vi "create.vi"(5 "Reference":string, 6 "Balance":dbl, 7 "Date":timestamp, 8 "error in (no error)":errorcluster, 9 "Category":string, 10 "Description":string, 11 "Amount":dbl) -> (0 "error out":errorcluster, 3 "Banking Transaction out":refnum<class "Banking Transaction.lvclass">)   [LabVIEW 2018, in "Banking Transaction.lvclass"]
uses:
  Banking Transaction.lvclass
  C:/GitRepos/Filthy-Lucre-Budgetizer/source/support/classes/Transaction/Transaction.lvclass
  Banking Transaction.lvclass/Banking Transaction.ctl
  Transaction/Transaction.lvclass
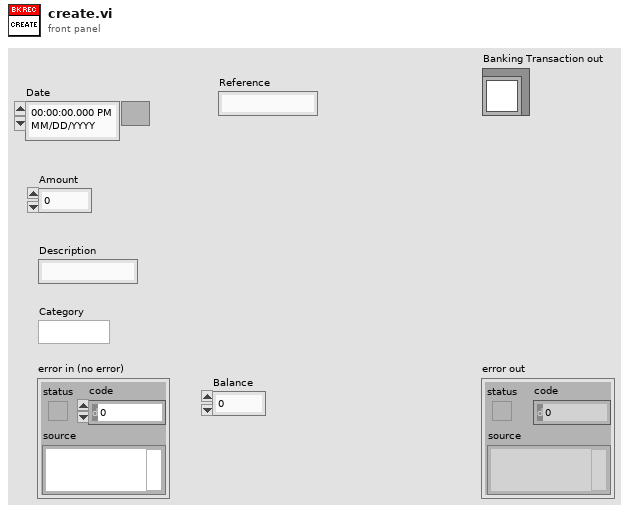
[diagram p1: front panel]
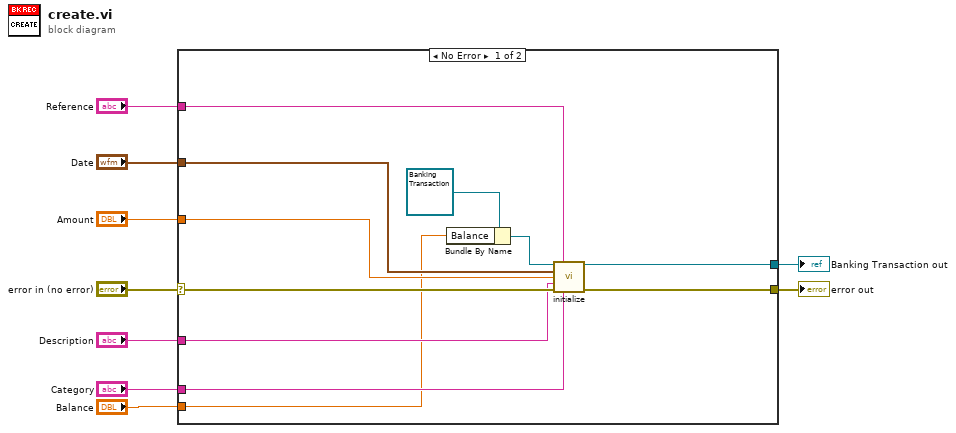
[diagram p0: block diagram]
diagram:
  n1 = case shown="No Error" "error in (no error)" {
    selector: "error in (no error)" -> [w19 w21]
    tunnel: [w18 w21] -> w8
    tunnel: [w20 _] -> w7
    tunnel: "Reference" -> [w15 _]
    tunnel: "Date" -> [w14 _]
    tunnel: "Amount" -> [w13 _]
    tunnel: "Description" -> [w12 _]
    tunnel: "Category" -> [w11 _]
    tunnel: "Balance" -> [w10 _]
    frame No Error {
      n2 = Bundle By Name(cluster=refnum<class "Banking Transaction.lvclass"> refnum ("Banking Transaction in"), "Balance"=w10) -> (w16:refnum<class "Banking Transaction.lvclass">)
      n3 = call "initialize.vi"("Transaction in"=w16, "Reference"=w15, "Date"=w14, "Amount"=w13, "Description"=w12, "error in (no error)"=w19, "Category"=w11) -> ("Transaction out"=w20:refnum<class "Banking Transaction.lvclass">, "error out"=w18:errorcluster)  [unwired: 7 in]
    }
    frame Error {
    }
  }
  "error out" <- w8
  "Banking Transaction out" <- w7
